vi "global_eco.vi"   [LabVIEW 2015]
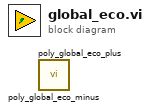
[diagram p0: block diagram]
diagram:
  n1 = call "poly_global_eco_minus.vi"() -> ()  [unwired: 5 in, 1 out]
  n2 = call "poly_global_eco_plus.vi"() -> ()  [unwired: 5 in, 1 out]
